vi "rapid_temp_control.vi"() -> ()   [LabVIEW 2009]
uses:
  <vilib>/DAQmx/create/timing.llb/DAQmx Create Timing Source.vi
  <vilib>/DAQmx/create/timing.llb/DAQmx Create Timing Source (Control Loop From Task).vi
  <vilib>/Platform/TimedLoop/XDataNode/XDataNode.xnode
  <vilib>/Platform/TimedLoop/XDataNode/loadlvalarms.vi
  <vilib>/Platform/TimedLoop/XDataNode/timing_clust.ctl
  <vilib>/Platform/TimedLoop/XDataNode/nitl_modes.ctl
  <vilib>/Platform/TimedLoop/XDataNode/wakeup.ctl
  <vilib>/DAQmx/write.llb/DAQmx Write (Analog 2D DBL NChan NSamp).vi
  <vilib>/DAQmx/read.llb/DAQmx Read (Analog 1D DBL 1Chan NSamp).vi
  <vilib>/Platform/TimedLoop/XDataNode/XDNodeRunTimeDep.lvlib
  <vilib>/Analysis/NI_AALBase.lvlib
panel:
  out "Measurement 2":dbl[][](graph) caption="Measurement"
  out "Tset":dbl
  out "Laser ON":bool
  out "Estimated temperature":dbl
  in  "Repeats":dbl=3.0 format="%0.0f"
  in  "Hysteresis [C]":dbl=3.0 format="%0.0f"
  in  "Max laser power [%]":dbl format="%0.0f"
  in  "Post wait  [ms]":dbl=1000.0 format="%0.2f"
  in  "Temperature \nhold time [ms]":dbl=100.0 format="%0.2f"
  in  "Pre wait  [ms]":dbl=1000.0 format="%0.2f"
  in  "Temperature jump (C)":dbl=10.0 format="%0.2f"
  in  "I0 [pA]":dbl format="%0.2f"
  in  "T0 [C]":dbl=25.0 format="%0.2f"
  in  "Minimum Value":dbl=-5.0 caption="AI Minimum Value" format="%0.2f"
  in  "Maximum Value":dbl=5.0 caption="AI Maximum Value" format="%0.2f"
  in  "Electrode voltage [mV]":dbl format="%0.2f"
  in  "Ea [J/mol]":dbl=3.4 format="%0.2f"
  out "Running":bool
  in  "exit":bool
  in  "Run mode":T1(ring)
  out "Measurement":dbl[](graph)
  in  "rate":dbl=1000.0 format="%0.2f"
  in  "stop":bool
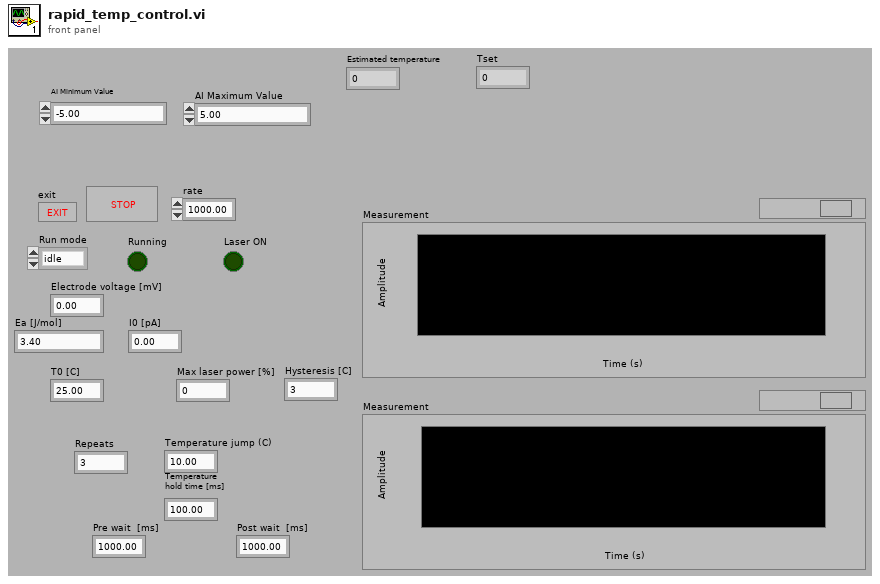
[diagram p1: front panel]
types:
  T1 = enum16{"idle", "generate protocol", "record electrophysiology"}
  T2 = typedef "XDNodeRunTimeDep.lvlib/timing_clust.ctl" = cluster{"Expected End [f-1]":u64, "Actual End [f-1]":u64, "Finished Late? [f-1]":bool, "Expected End [i-1]":u64, "Actual End [i-1]":u64, "Finished Late? [i-1]":bool, "Expected Start [i]":u64, "Actual Start [i]":u64, "Expected Start [f]":u64, "Actual Start [f]":u64, "Source Name":string, "Structure Name":string, "Period":i64, "Deadline":i64, "Offset":i64, "Start":i64, "Priority":i32, "Timeout":i32, "Mode":T3, "Wakeup Reason":T4, "Error":errorcluster, "Source Type":string, "Secondary Source Type":string, "Global End Time":u64, "Global Start Time":u64, "Frame Duration":u64, "Iteration Duration":u64, "Assigned CPU":i32, "I/O Scan Engine Mode":u32}
  T3 = typedef "XDNodeRunTimeDep.lvlib/nitl_modes.ctl" = enum32{"No Change", "Process missed periods, maintain original phase", "Discard missed periods, maintain original phase", "Process missed periods, ignore original phase", "Discard missed periods, ignore original phase"}
  T4 = typedef "XDNodeRunTimeDep.lvlib/wakeup.ctl" = enum32{"Normal", "Aborted", "Asynchronous wakeup", "Timing source error", "Timed loop error", "Timeout"}
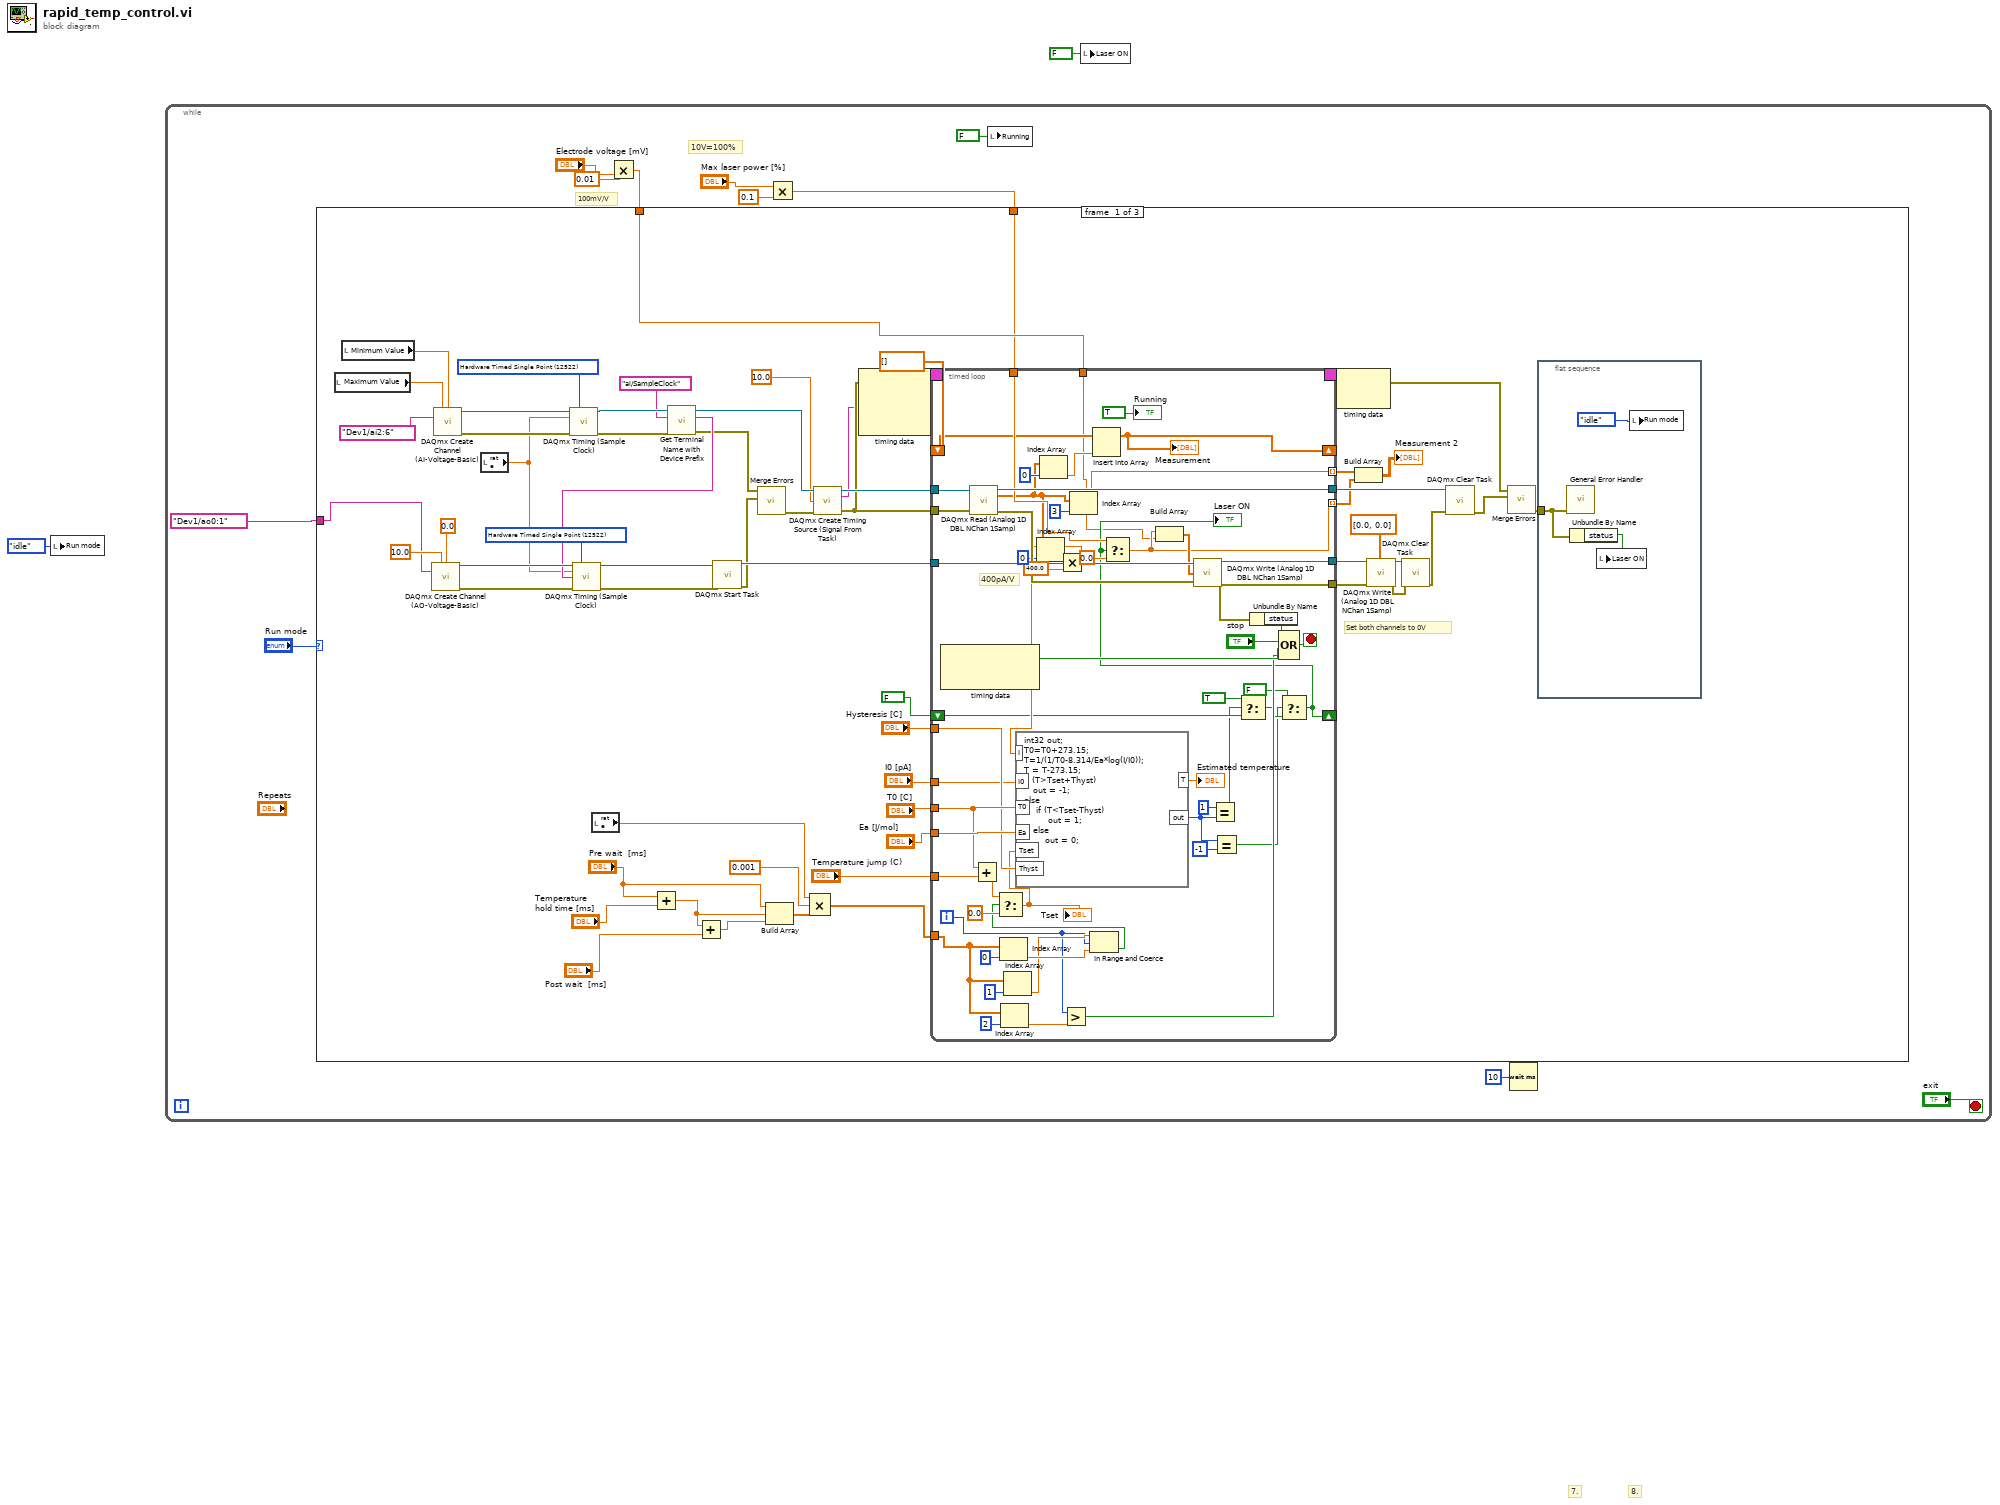
[diagram p0: block diagram]
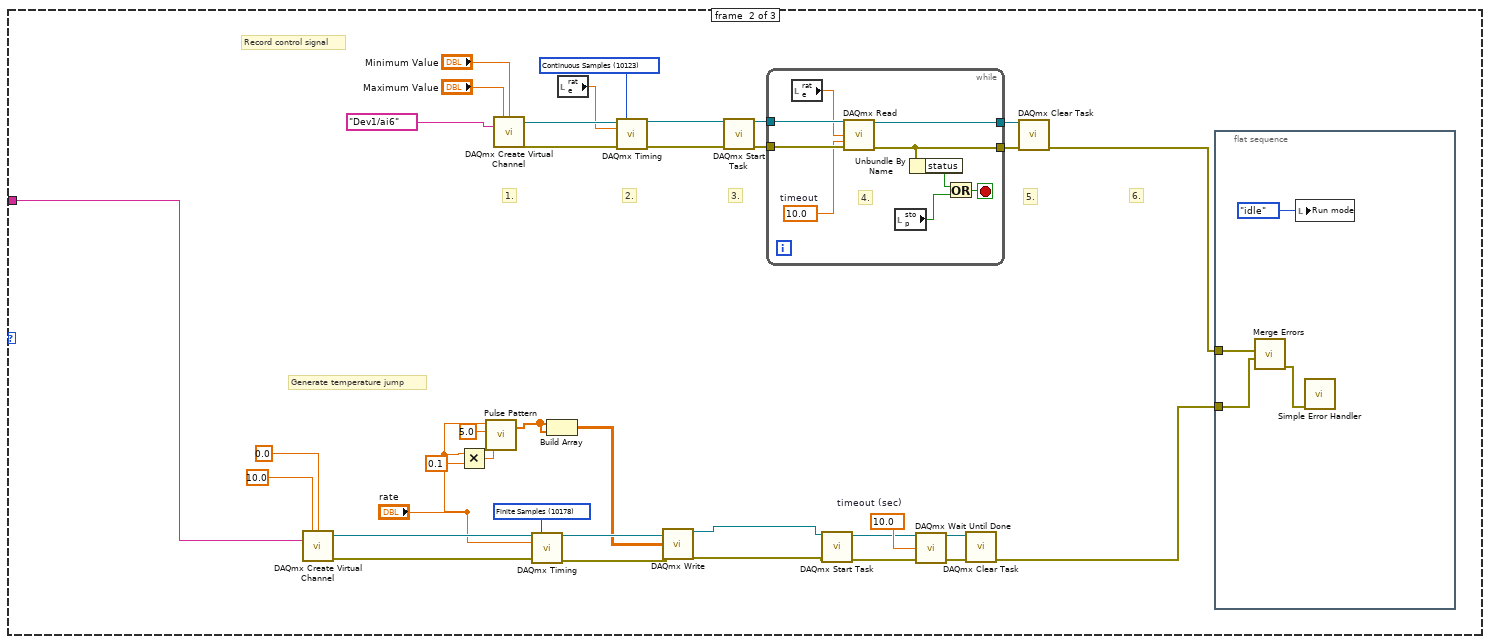
[diagram p2: hidden frame]
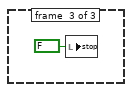
[diagram p3: hidden frame]
diagram:
  # "7."
  # "8."
  n1 = local write "Run mode"(T1."idle" ("Run mode")) -> ()
  n2 = while {
    stop <- "exit" stop-if-true
    # "10V=100%"
    # "100mV/V"
    n3 = Multiply(x=0.01 ("y"), y="Electrode voltage [mV]") -> (x*y=w6:dbl)
    n4 = Multiply(x="Max laser power [%]", y=0.1) -> (x*y=w3:dbl)
    n5 = case shown="\"generate protocol\"" "Run mode" {
      tunnel: tag "Dev1/ao0:1" ("Physical Channels") -> [w42 w164 _]
      tunnel: w6 -> [w41 _ _]
      tunnel: w3 -> [w33 _ _]
      frame #0 {
        w61 = 12522 items=["Finite Samples"=10178, "Continuous Samples"=10123, "Hardware Timed Single Point"=12522] ("sample mode")
        w62 = 12522 items=["Finite Samples"=10178, "Continuous Samples"=10123, "Hardware Timed Single Point"=12522] ("sample mode")
        # "Set both channels to 0V"
        n6 = local read "Maximum Value"() -> (w35:dbl)
        n7 = local read "Minimum Value"() -> (w34:dbl)
        n8 = call-poly <vilib>:"DAQmx Create Channel (AO-Voltage-Basic).vi"("maximum value"=10.0 ("Maximum Value"), "minimum value"=0.0 ("Minimum Value"), "physical channels"=w42) -> ("task out"=w67:refnum<k21>, "error out"=w66:errorcluster)  [unwired: 11 in]
        n9 = call-poly <vilib>:"DAQmx Create Channel (AI-Voltage-Basic).vi"("maximum value"=w35, "minimum value"=w34, "physical channels"=tag "Dev1/ai2:6" ("Physical Channels 2")) -> ("task out"=w70:refnum<k21>, "error out"=w71:errorcluster)  [unwired: 11 in]
        n10 = local read "rate"() -> (w43:dbl)
        n11 = call-poly <vilib>:"DAQmx Timing (Sample Clock).vi"("task/channels in"=w70, "sample mode"=w62, "rate"=w43, "error in"=w71) -> ("task out"=w52:refnum<k21>, "error out"=w49:errorcluster)  [unwired: 10 in]
        n12 = local read "rate"() -> (w23:dbl)
        n13 = Add(x="Pre wait  [ms]", y="Temperature \nhold time [ms]") -> (x+y=w26:dbl)
        n14 = call "Get Terminal Name with Device Prefix.vi"("error in (no error)"=w49, "Local Terminal Name"="ai/SampleClock", "task/channels in"=w52) -> ("error out"=w48:errorcluster, "Terminal Name with Device Prefix"=w50:tag, "task out"=w51:refnum<k21>)  [unwired: 6 in]
        n15 = call-poly <vilib>:"DAQmx Timing (Sample Clock).vi"("task/channels in"=w67, "sample mode"=w61, "rate"=w43, "source"=w50, "error in"=w66) -> ("task out"=w47:refnum<k21>, "error out"=w46:errorcluster)  [unwired: 9 in]
        n16 = Add(x=w26, y="Post wait  [ms]") -> (x+y=w27:dbl)
        n17 = call <vilib>:"DAQmx Start Task.vi"("task/channels in"=w47, "error in"=w46) -> ("task out"=w65:refnum<k21>, "error out"=w63:errorcluster)  [unwired: 12 in]
        n18 = call <vilib>:"Merge Errors.vi"("error in 2 (no error)"=w63, "error in 1 (no error)"=w48) -> ("error out"=w60:errorcluster)  [unwired: 5 in]
        n19 = Build Array("Pre wait  [ms]", w26, w27) -> (w24:dbl[])
        n20 = Compound Arithmetic op=MULTIPLY(w23, 0.001 ("Temperature jump (C)"), w24) -> (w21:dbl[])
        n21 = call-poly "DAQmx Create Timing Source (Signal From Task).vi"("task/channels in"=w51, "sleep time (us)"=10.0, "error in"=w60) -> ("task out"=w59:refnum<k21>, "timing source out"=w54:string, "error out"=w55:errorcluster)  [unwired: 10 in]
        n22 = node-c288(w55, w54) -> (w74:T2)  [unwired: 1 in]
        n23 = timed-loop {
          timing-out: [_] -> w73
          timing: w74 -> [_]
          tunnel: [w125] -> w39
          tunnel: w55 -> [w130]
          tunnel: w59 -> [w131]
          tunnel: [w132] -> w40
          tunnel: w65 -> [w133]
          tunnel: [w134] -> w72
          shift-right: [w120] -> _
          shift-left: dbl[] [] -> [w85]
          tunnel: w41 -> [w78]
          tunnel: w33 -> [w115]
          tunnel: "I0 [pA]" -> [w84]
          tunnel: "T0 [C]" -> [w111]
          tunnel: "Ea [J/mol]" -> [w113]
          tunnel: w21 -> [w103]
          tunnel: "Temperature jump (C)" -> [w112]
          tunnel: "Hysteresis [C]" -> [w98]
          shift-right: [w86] -> _
          shift-left: FALSE ("x = y?") -> [w95]
          tunnel: [w80] -> w15 mode=indexing
          tunnel: [w79] -> w16 mode=indexing
          i -> [w101]
          stop <- w128 stop-if-true
          # "400pA/V"
          n24 = node-c288() -> (w124:bool)  [unwired: 1 in, 1 out]
          n25 = call-poly <vilib>:"DAQmx Read (Analog 1D DBL NChan 1Samp).vi"("task/channels in"=w131, "error in"=w130) -> ("task out"=w134:refnum<k21>, "data"=w83:dbl[], "error out"=w126:errorcluster)  [unwired: 11 in]
          n26 = Add(x=w111, y=w112) -> (x+y=w110:dbl)
          n27 = Index Array(array=w103, index=0) -> (element=w108:dbl)
          n28 = Index Array(array=w103, index=2) -> (element=w100:dbl)
          n29 = Index Array(array=w103, index=1) -> (element=w105:dbl)
          n30 = Index Array(array=w83, index=0) -> (element=w123:dbl)
          n31 = Index Array(array=w83, index=0) -> (element=w81:dbl)
          n32 = Multiply(x=w123, y=400.0) -> (x*y=w116:dbl)
          n33 = Greater?(x=w101, y=w100) -> (0:w99:bool)
          n34 = Index Array(array=w83, index=3) -> (element=w80:dbl)
          n35 = In Range and Coerce(upper limit=w105, x=w101, lower limit=w108) -> (In Range?=w104:bool)  [unwired: 1 out]
          n36 = Select(t=w110, s=w104, f=0.0) -> (s? t:f=w87:dbl)
          "Tset" <- w87
          n37 = formula code="int32 out;\nT0=T0+273.15;\nT=1/(1/T0-8.314/Ea*log(I/I0));\nT = T-273.15;\nif (T>Tset+Thyst)    \n   out = -1;\nelse\n    if (T<Tset-Thyst)    \n        out = 1;\n   else\n       out = 0;"("I"=w116, "I0"=w84, "T0"=w111, "Ea"=w113, "Thyst"=w98, "Tset"=w87) -> ("T"=→"Estimated temperature":dbl, "out"=w92:i32)
          n38 = Insert Into Array(array=w85, new element=w81) -> (w120:dbl[])  [unwired: 1 in]
          "Measurement" <- w120
          n39 = Equal?(x=1, y=w92) -> (x = y?=w93:bool)
          n40 = Equal?(x=w92, y=-1) -> (x = y?=w89:bool)
          n41 = Select(t=TRUE, s=w93, f=w95) -> (s? t:f=w90:bool)
          n42 = Select(t=FALSE, s=w89, f=w90) -> (s? t:f=w86:bool)
          "Laser ON" <- w86
          n43 = Select(t=w115, s=w86, f=0.0) -> (s? t:f=w79:dbl)
          n44 = Build Array(w79, w78) -> (w118:dbl[])
          n45 = call-poly <vilib>:"DAQmx Write (Analog 1D DBL NChan 1Samp).vi"("task/channels in"=w133, "data"=w118, "error in"=w126) -> ("task out"=w132:refnum<k21>, "error out"=w125:errorcluster)  [unwired: 10 in, 1 out]
          n46 = Unbundle By Name(w125) -> ("status"=w129:bool)
          n47 = Compound Arithmetic op=OR(w129, "stop", w124, w99) -> (w128:bool)
          "Running" <- TRUE ("Running")
        }
        n48 = node-c288(w73) -> (w53:errorcluster)
        n49 = Build Array(w15, w16) -> (→"Measurement 2":dbl[][])
        n50 = call-poly <vilib>:"DAQmx Write (Analog 1D DBL NChan 1Samp).vi"("task/channels in"=w40, "data"=dbl[] [0.0, 0.0], "error in"=w39) -> ("task out"=w38:refnum<k21>, "error out"=w36:errorcluster)  [unwired: 10 in, 1 out]
        n51 = call <vilib>:"DAQmx Clear Task.vi"("task in"=w38, "error in"=w36) -> ("error out"=w58:errorcluster)  [unwired: 13 in]
        n52 = call <vilib>:"DAQmx Clear Task.vi"("task in"=w72, "error in"=w58) -> ("error out"=w57:errorcluster)  [unwired: 13 in]
        n53 = call <vilib>:"Merge Errors.vi"("error in 2 (no error)"=w57, "error in 1 (no error)"=w53) -> ("error out"=w56:errorcluster)  [unwired: 5 in]
        n54 = flat-sequence {
          tunnel: w56 -> [w76]
          frame #0 {
            n55 = call <vilib>:"General Error Handler.vi"("error in (no error)"=w76) -> ()  [unwired: 10 in, 5 out]
            n56 = Unbundle By Name(w76) -> ("status"=w75:bool)
            n57 = local write "Laser ON"(w75) -> ()
            n58 = local write "Run mode"(T1."idle" ("Run mode")) -> ()
          }
        }
      }
      frame #1 {
        w148 = 10123 items=["Finite Samples"=10178, "Continuous Samples"=10123] ("sample mode")
        w175 = 10.0  # timeout (sec)
        w165 = 10178 items=["Finite Samples"=10178, "Continuous Samples"=10123] ("sample mode")
        # "6."
        # "5."
        # "3."
        # "2."
        # "1."
        # "Record control signal"
        # "Generate temperature jump"
        n59 = call-poly <vilib>:"DAQmx Create Virtual Channel.vi"("maximum value"=10.0 ("Maximum Value"), "minimum value"=0.0 ("Minimum Value"), "physical channels"=w164) -> ("task out"=w178:refnum<k21>, "error out"=w179:errorcluster)  [unwired: 11 in]
        n60 = Multiply(x="rate", y=0.1) -> (x*y=w162:dbl)
        n61 = call <vilib>:"Pulse Pattern.vi"("width"=w162, "amplitude"=5.0, "samples"="rate") -> ("Pulse Pattern"=w158:dbl[])  [unwired: 1 in, 1 out]
        n62 = call-poly <vilib>:"DAQmx Create Virtual Channel.vi"("maximum value"="Maximum Value", "minimum value"="Minimum Value", "physical channels"=tag "Dev1/ai6" ("Physical Channel")) -> ("task out"=w152:refnum<k21>, "error out"=w154:errorcluster)  [unwired: 11 in]
        n63 = call-poly <vilib>:"DAQmx Timing.vi"("task/channels in"=w178, "sample mode"=w165, "rate"="rate", "error in"=w179) -> ("task out"=w168:refnum<k21>, "error out"=w169:errorcluster)  [unwired: 10 in]
        n64 = Build Array(w158, w158) -> (w159:dbl[][])
        n65 = local read "rate"() -> (w144:dbl)
        n66 = call-poly <vilib>:"DAQmx Timing.vi"("task/channels in"=w152, "sample mode"=w148, "rate"=w144, "error in"=w154) -> ("task out"=w147:refnum<k21>, "error out"=w146:errorcluster)  [unwired: 10 in]
        n67 = call-poly <vilib>:"DAQmx Write.vi"("task/channels in"=w168, "data"=w159, "error in"=w169) -> ("task out"=w176:refnum<k21>, "error out"=w177:errorcluster)  [unwired: 10 in, 1 out]
        n68 = call <vilib>:"DAQmx Start Task.vi"("task/channels in"=w147, "error in"=w146) -> ("task out"=w151:refnum<k21>, "error out"=w153:errorcluster)  [unwired: 12 in]
        n69 = while {
          tunnel: w153 -> [w188]
          tunnel: w151 -> [w187]
          tunnel: [w186] -> w150
          tunnel: [w185] -> w145
          stop <- w183 stop-if-true
          w182 = 10.0  # timeout
          # "4."
          n70 = local read "rate"() -> (w181:dbl)
          n71 = call-poly <vilib>:"DAQmx Read.vi"("task/channels in"=w187, "number of samples per channel"=w181, "timeout"=w182, "error in"=w188) -> ("task out"=w186:refnum<k21>, "error out"=w185:errorcluster)  [unwired: 9 in, 1 out]
          n72 = local read "stop"() -> (w180:bool)
          n73 = Unbundle By Name(w185) -> ("status"=w184:bool)
          n74 = Or(x=w184, y=w180) -> (x .or. y?=w183:bool)
        }
        n75 = call <vilib>:"DAQmx Start Task.vi"("task/channels in"=w176, "error in"=w177) -> ("task out"=w170:refnum<k21>, "error out"=w171:errorcluster)  [unwired: 12 in]
        n76 = call <vilib>:"DAQmx Wait Until Done.vi"("task/channels in"=w170, "timeout (sec)"=w175, "error in"=w171) -> ("task out"=w174:refnum<k21>, "error out"=w173:errorcluster)  [unwired: 11 in]
        n77 = call <vilib>:"DAQmx Clear Task.vi"("task in"=w174, "error in"=w173) -> ("error out"=w172:errorcluster)  [unwired: 13 in]
        n78 = call <vilib>:"DAQmx Clear Task.vi"("task in"=w150, "error in"=w145) -> ("error out"=w157:errorcluster)  [unwired: 13 in]
        n79 = flat-sequence {
          tunnel: w172 -> [w191]
          tunnel: w157 -> [w190]
          frame #0 {
            n80 = call <vilib>:"Merge Errors.vi"("error in 3 (no error)"=w191, "error in 2 (no error)"=w190) -> ("error out"=w189:errorcluster)  [unwired: 5 in]
            n81 = local write "Run mode"(T1."idle" ("Run mode")) -> ()
            n82 = call <vilib>:"Simple Error Handler.vi"("error in (no error)"=w189) -> ()  [unwired: 4 in, 5 out]
          }
        }
      }
      frame #2 {
        n83 = local write "stop"(FALSE ("stop")) -> ()
      }
    }
    n84 = local write "Running"(FALSE ("Running")) -> ()
    n85 = Wait (ms)(milliseconds to wait=u32 10) -> ()  [unwired: 1 out]
  }
  n86 = local write "Laser ON"(FALSE ("Laser ON")) -> ()
